vi "Drive Turbo.vi"(4 "Slow Rotation":bool, 6 "Turbo":bool, 9 "Z":dbl, 10 "Y":dbl, 11 "X":dbl) -> (1 "Z 2":dbl, 2 "Y 2":dbl, 3 "X 2":dbl)   [LabVIEW 2017]
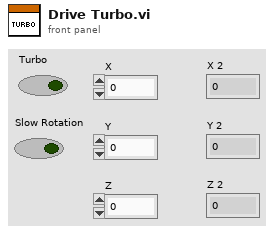
[diagram p1: front panel]
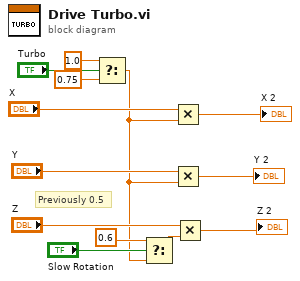
[diagram p0: block diagram]
diagram:
  # "Previously 0.5"
  n1 = Select(t=1.0, s="Turbo", f=0.75) -> (s? t:f=w1:dbl)
  n2 = Select(t=0.6, s="Slow Rotation", f=w1) -> (s? t:f=w3:dbl)
  n3 = Multiply(x="X", y=w1) -> (x*y=→"X 2":dbl)
  n4 = Multiply(x="Y", y=w1) -> (x*y=→"Y 2":dbl)
  n5 = Multiply(x="Z", y=w3) -> (x*y=→"Z 2":dbl)
